vi "Continue Acquisition.vi"(8 "error in (no error)":errorcluster, 10 "Data Buffer":T1, 11 "TDMS Data Source in":refnum<class "TDMS Data Source.lvclass">) -> (0 "error out":errorcluster, 3 "TDMS Data Source out":refnum<class "TDMS Data Source.lvclass">)   [LabVIEW 2020, in "TDMS Data Source.lvlib" / "TDMS Data Source.lvclass"]
uses:
  TDMS Data Source.lvclass
  C:/Users/natan/Documents/G2CPU-Performance-Demo/Data Source/Data Source/Data Source.lvclass
  C:/Program Files/National Instruments/LabVIEW 2026/vi.lib/ActorFramework/Actor/Actor.lvclass
  GPU FFT Calculator/GPU FFT Calculator/Data Source Buffer.ctl
  <vilib>/ActorFramework/Actor/Actor.lvclass/Actor.ctl
  <vilib>/ActorFramework/Message Enqueuer/Message Enqueuer.lvclass/Message Enqueuer.ctl
  TDMS Data Source Messages/Start Reading File Msg/Start Reading File Msg.lvclass/Start Reading File Msg.ctl
  <vilib>/ActorFramework/Message Enqueuer/Init from Existing Queue.vi
  <vilib>/ActorFramework/Message Enqueuer/Enqueue.vi
  TDMS Data Source Messages/Start Reading File Msg/Start Reading File Msg.lvclass
  C:/Program Files/National Instruments/LabVIEW 2026/vi.lib/ActorFramework/Message/Message.lvclass
  <vilib>/ActorFramework/Message Priority Queue/Priority Enqueue.vi
  <vilib>/ActorFramework/Message Enqueuer/Message Enqueuer.lvclass
  Data Source/Data Source/Data Source.lvclass
  <vilib>/ActorFramework/Actor/Actor.lvclass
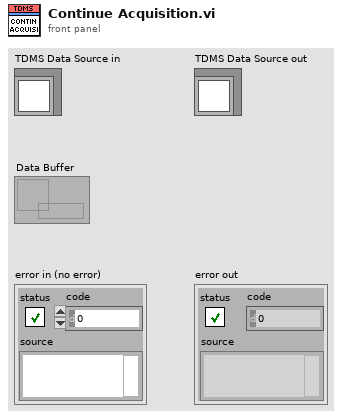
[diagram p1: front panel]
types:
  T1 = typedef "Data Source.lvlib/Data Source.lvclass/Data Source Buffer.ctl" = refnum<data-value>
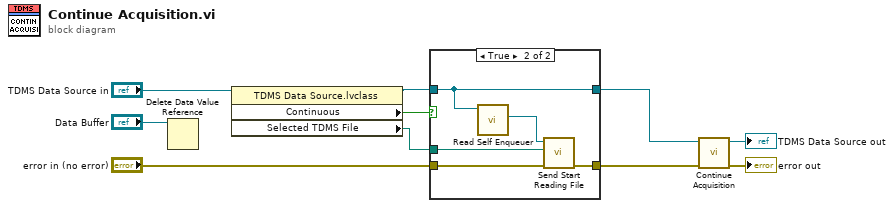
[diagram p0: block diagram]
diagram:
  n1 = Delete Data Value Reference(data value reference="Data Buffer") -> ()  [unwired: 1 in, 2 out]
  n2 = property on="Property Node" class="TDMS Data Source.lvclass"(reference="TDMS Data Source in") -> (reference out=w8:refnum<class "TDMS Data Source.lvclass">, "Continuous"=w7:bool, "Selected TDMS File"=w6:path)  [unwired: 1 in, 1 out]
  n3 = case shown="True" w7 {
    tunnel: "error in (no error)" -> [w11 w14]
    tunnel: [w12 w17] -> w5
    tunnel: w8 -> [w12 w17]
    tunnel: w6 -> [_ w15]
    tunnel: [w11 w13] -> w4
    frame False {
    }
    frame True {
      n4 = call <vilib>:"Read Self Enqueuer.vi"("Actor"=w17) -> ("Self Enqueuer"=w16:refnum<class "Message Enqueuer.lvclass">)  [unwired: 10 in]
      n5 = call "Send Start Reading File.vi"("error in (no error)"=w14, "TDMS File"=w15, "Message Enqueuer"=w16) -> ("error out"=w13:errorcluster)  [unwired: 7 in, 1 out]
    }
  }
  n6 = call-parent "Continue Acquisition.vi"("error in (no error)"=w4, "Data Source in"=w5) -> ("error out"=→"error out":errorcluster, "Data Source out"=→"TDMS Data Source out":refnum<class "TDMS Data Source.lvclass">)  [unwired: 8 in]
